vi "SimpleNDL8example.vi"() -> ()   [LabVIEW 2024]
panel:
  out "AND CC":dbl=14.609375 format="%#12.0f"
  out "AND":dbl=14.609375 format="%#12.0f"
  out "# Ereignisse 2":dbl=14.609375 format="%#12.0f"
  out "# Ereignisse":dbl=14.609375 format="%#12.0f"
  out "Versoion":string
  out "NemBox ID":string
  in  "Stop":bool=TRUE
  out "Zeit seit Start [s]":dbl=14.609375 format="%#12.0f"
  out "Zaehlrate (Hz)":dbl=14.609375 format="%#12.2f"
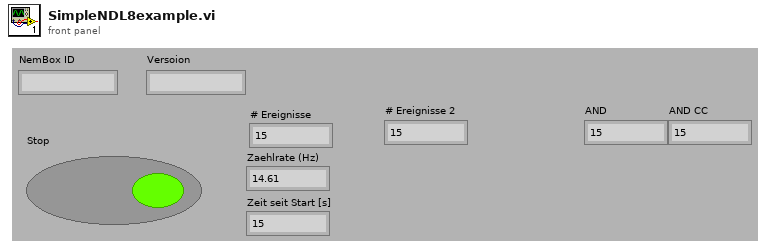
[diagram p1: front panel]
types:
  T1 = enum16{"Connect", "Get IN", "Write Threshold", "Write Hysteresis", "Write Stretch"}
  T2 = enum16{"Connect", "Set A", "Set B", "Set C", "Set D", "Set E", "Set F", "Set G", "Set H", "Get AND", "Read Counter", "Clear Counter"}
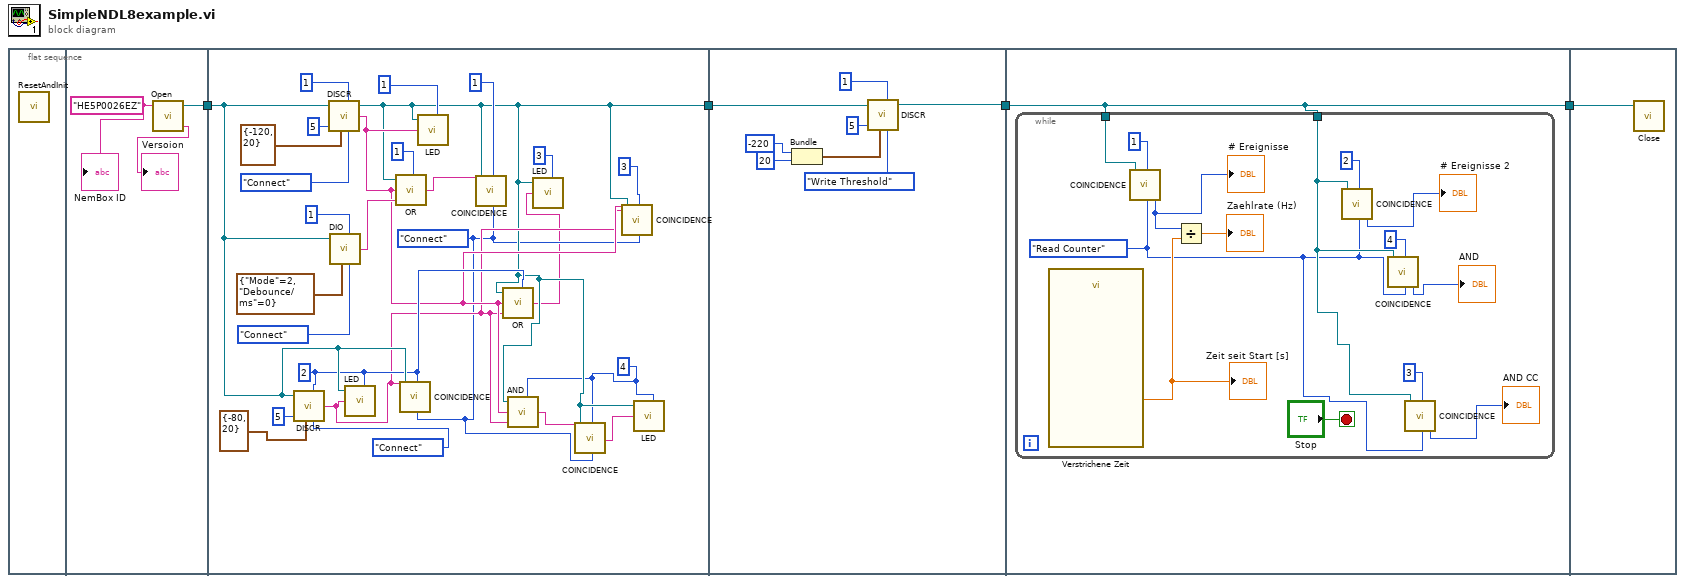
[diagram p0: block diagram]
diagram:
  n1 = flat-sequence {
    tunnel: [w7] -> w3
    tunnel: w3 -> [w21]
    tunnel: [w14] -> w2
    tunnel: w2 -> [w40]
    tunnel: [w39] -> w1
    tunnel: [w43] -> w4
    tunnel: w1 -> [w43]
    tunnel: w4 -> [w58]
    frame #0 {
      n2 = call <userlib>:"ResetAndInit.vi"() -> ()  [unwired: 1 out]
    }
    frame #1 {
      w6 = "HE5P0026EZ"
      n3 = call <userlib>:"Open.vi"("USB_LogicBox"=w6) -> ("USB Out"=w7:refnum<visa-resource-name>, "Version"=→"Versoion":string)  [unwired: 1 in, 6 out]
      "NemBox ID" <- w6
    }
    frame #2 {
      w10 = 4
      w20 = 2
      w13 = T2."Connect"
      n4 = call <userlib>:"DISCR.vi"("USB In"=w21, "Stretch/10ns"=u8 5, "Params"=cluster{i32, i32} {-80, 20} ("Schwelle"), "DISCR#"=w20, "Function"=T1."Connect") -> ("DISCR"=w15:string)  [unwired: 4 out]
      n5 = call <userlib>:"DISCR.vi"("USB In"=w21, "Stretch/10ns"=u8 5, "Params"=cluster{i32, i32} {-120, 20} ("Schwelle"), "DISCR#"=1, "Function"=T1."Connect") -> ("USB Out"=w14:refnum<visa-resource-name>, "DISCR"=w16:string)  [unwired: 3 out]
      n6 = call <userlib>:"DIO.vi"("USB In"=w21, "Params"=cluster{"Mode":u8, "Debounce/ms":u8} {"Mode"=2, "Debounce/ms"=0}, "DIO#"=1, "Function"=enum16{"Connect", "Set DO", "Get DI"}."Connect") -> ("DI"=w27:string)  [unwired: 1 in, 4 out]
      n7 = call <userlib>:"LED.vi"("USB In"=w21, "STATE"=w15, "LED#"=w20) -> ()  [unwired: 1 in, 6 out]
      n8 = call <userlib>:"OR.vi"("USB In"=w14, "A"=w16, "B"=w27, "LOGIC#"=1) -> ("OR"=w25:string)  [unwired: 1 in, 4 out]
      n9 = call <userlib>:"COINCIDENCE.vi"("A"=w15, "USB In"=w21, "CC#"=w20, "Function"=w13) -> ()  [unwired: 7 in, 17 out]
      n10 = call <userlib>:"LED.vi"("USB In"=w14, "STATE"=w16, "LED#"=1) -> ()  [unwired: 1 in, 6 out]
      n11 = call <userlib>:"COINCIDENCE.vi"("A"=w25, "USB In"=w14, "CC#"=1, "Function"=w13) -> ()  [unwired: 7 in, 17 out]
      n12 = call <userlib>:"OR.vi"("USB In"=w14, "A"=w16, "B"=w15, "LOGIC#"=w20) -> ("OR"=w11:string)  [unwired: 1 in, 4 out]
      n13 = call <userlib>:"AND.vi"("USB In"=w14, "A"=w16, "B"=w15, "LOGIC#"=w10) -> ("AND"=w19:string)  [unwired: 4 in, 1 out]
      n14 = call <userlib>:"LED.vi"("USB In"=w14, "STATE"=w11, "LED#"=3) -> ()  [unwired: 1 in, 6 out]
      n15 = call <userlib>:"COINCIDENCE.vi"("A"=w19, "USB In"=w14, "CC#"=w10, "Function"=w13) -> ("AND"=w18:string)  [unwired: 7 in, 16 out]
      n16 = call <userlib>:"COINCIDENCE.vi"("A"=w16, "B"=w15, "USB In"=w14, "CC#"=3, "Function"=w13) -> ()  [unwired: 6 in, 17 out]
      n17 = call <userlib>:"LED.vi"("USB In"=w14, "STATE"=w18, "LED#"=w10) -> ()  [unwired: 1 in, 6 out]
    }
    frame #3 {
      n18 = Bundle(-220, 20) -> (w37:cluster{i32, i32})  [unwired: 1 out]
      n19 = call <userlib>:"DISCR.vi"("USB In"=w40, "Stretch/10ns"=u8 5, "Params"=w37, "DISCR#"=1, "Function"=T1."Write Threshold") -> ("USB Out"=w39:refnum<visa-resource-name>)  [unwired: 4 out]
    }
    frame #4 {
      n20 = while {
        tunnel: w43 -> [w53]
        tunnel: w43 -> [w45]
        stop <- "Stop" stop-if-true
        w44 = T2."Read Counter"
        n21 = call "Verstrichene Zeit"() -> ("Elapsed Time (s)"=w55:dbl)  [unwired: 5 in, 14 out]
        "Zeit seit Start [s]" <- w55
        n22 = call <userlib>:"COINCIDENCE.vi"("USB In"=w53, "CC#"=1, "Function"=w44) -> ("Counter"=w52:u32)  [unwired: 8 in, 16 out]
        "# Ereignisse" <- w52
        n23 = Divide(x=w52, y=w55) -> (x/y=→"Zaehlrate (Hz)":dbl)
        n24 = call <userlib>:"COINCIDENCE.vi"("USB In"=w45, "CC#"=2, "Function"=w44) -> ("Counter"=→"# Ereignisse 2":u32)  [unwired: 8 in, 16 out]
        n25 = call <userlib>:"COINCIDENCE.vi"("USB In"=w45, "CC#"=4, "Function"=w44) -> ("Counter"=→"AND":u32)  [unwired: 8 in, 16 out]
        n26 = call <userlib>:"COINCIDENCE.vi"("USB In"=w45, "CC#"=3, "Function"=w44) -> ("Counter"=→"AND CC":u32)  [unwired: 8 in, 16 out]
      }
    }
    frame #5 {
      n27 = call <userlib>:"Close.vi"("USB In"=w58) -> ()  [unwired: 1 in, 8 out]
    }
  }
